vi "roboRIO v1.0 Build MUX Configuration AO.vi"(11 "AO Channels List":T4) -> (3 "Channel Reservation Info":T1)   [LabVIEW 2021]
uses:
  <vilib>/myRIO/Common/Instrument Driver Framework/myRIO v1.0/AO/typedefs/AO Channels List.ctl
  <vilib>/myRIO/Common/Instrument Driver Framework/myRIO v1.0/AO/typedefs/AO Channels Enum.ctl
  <vilib>/myRIO/Common/Instrument Driver Framework/roboRIO v1.0/Resource Manager/typedefs/roboRIO v1.0 Channel Reservation List.ctl
  <vilib>/myRIO/Common/Instrument Driver Framework/roboRIO v1.0/Resource Manager/typedefs/roboRIO v1.0 Channel Reservation Info.ctl
  <vilib>/myRIO/Common/Instrument Driver Framework/roboRIO v1.0/Resource Manager/typedefs/roboRIO v1.0 Connector List.ctl
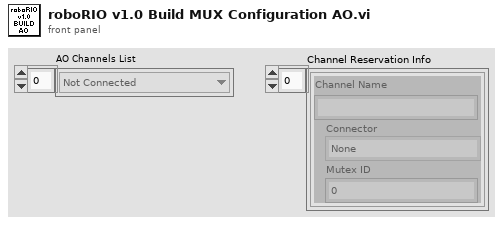
[diagram p1: front panel]
types:
  T1 = typedef "roboRIO v1.0 Channel Reservation List.ctl" = T2[]
  T2 = typedef "roboRIO v1.0 Channel Reservation Info.ctl" = cluster{"Channel Name":string, "Connector":T3, "Mutex ID":i32}
  T3 = typedef "roboRIO v1.0 Connector List.ctl" = enum32{"None", "ConnectorB", "ConnectorI2C", "ConnectorDIO", "ConnectorRSL", "ConnectorRELAY", "ConnectorAI", "ConnectorPWM", "ConnectorSPI"}
  T4 = typedef "AO Channels List.ctl" = T5[]
  T5 = typedef "AO Channels Enum.ctl" = enum16{"Not Connected", "AudioOut/Left", "AudioOut/Right", "C/AO0", "C/AO1", "A/AO0", "A/AO1", "B/AO0", "B/AO1"}
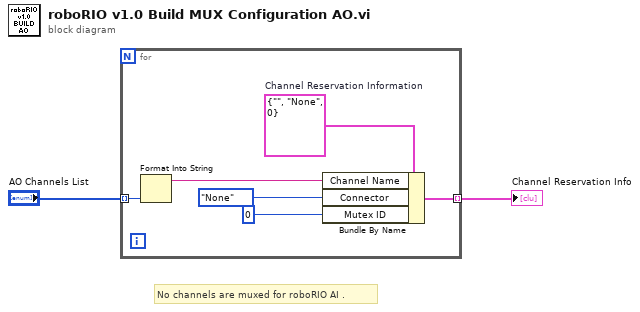
[diagram p0: block diagram]
diagram:
  # "No channels are muxed for roboRIO AI ."
  n1 = for {
    tunnel: "AO Channels List" -> [w5] mode=indexing
    tunnel: [w6] -> w1 mode=indexing
    w8 = T2 {"Channel Name"="", "Connector"=enum."None", "Mutex ID"=0}  # Channel Reservation Information
    n2 = Format Into String(w5) -> (resulting string=w7:string)  [unwired: 3 in, 1 out]
    n3 = Bundle By Name(cluster=w8, "Channel Name"=w7, "Connector"=roboRIO_v1.0_Connector_List."None", "Mutex ID"=0 ("Bit")) -> (w6:T2)
  }
  "Channel Reservation Info" <- w1
